vi "有人WiFi模块扫描信息.vi"(8 "error in (no error)":errorcluster caption="错误输入（无错误）", 11 "扫描广播回复":string[](array[string])) -> (0 "error out":errorcluster caption="错误输出", 3 "模块IP与MAC":cluster{"IP":string, "MAC":string}[](array[cluster]))   [LabVIEW 2017]
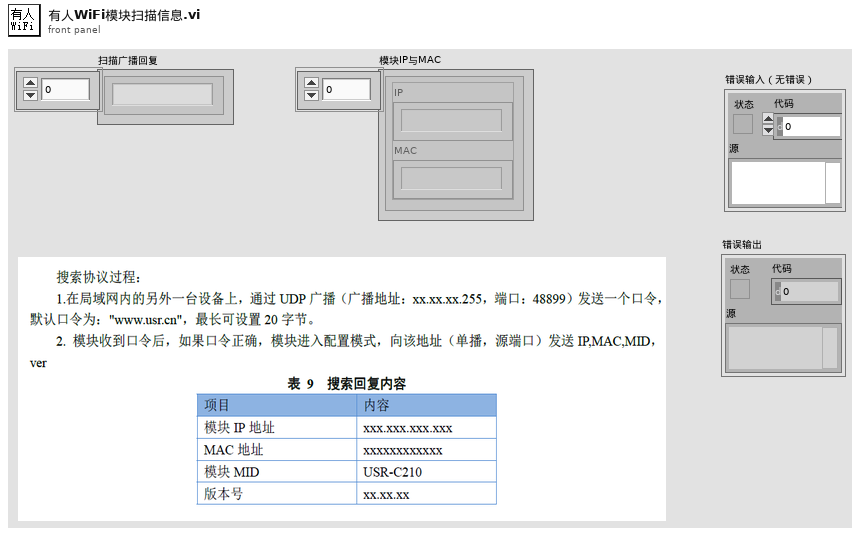
[diagram p1: front panel]
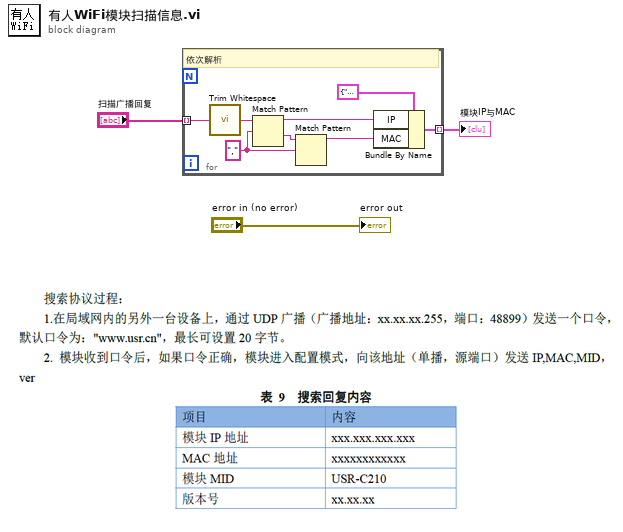
[diagram p0: block diagram]
diagram:
  n1 = for {
    tunnel: "扫描广播回复" -> [w11] mode=indexing
    tunnel: [w4] -> w2 mode=indexing
    w8 = "," ("正则表达式")
    # "依次解析"
    n2 = call <vilib>:"Trim Whitespace.vi"("string"=w11) -> ("trimmed string"=w10:string)  [unwired: 1 in]
    n3 = Match Pattern(string=w10, regular expression=w8) -> (before substring=w6:string, after substring=w9:string)  [unwired: 1 in, 2 out]
    n4 = Match Pattern(string=w9, regular expression=w8) -> (before substring=w5:string)  [unwired: 1 in, 3 out]
    n5 = Bundle By Name(cluster=cluster{"IP":string, "MAC":string} {"IP"="", "MAC"=""} ("输出簇"), "IP"=w6, "MAC"=w5) -> (w4:cluster{"IP":string, "MAC":string})
  }
  "模块IP与MAC" <- w2
  "error out" <- "error in (no error)"
